vi "MultiGrid_v2.vi"() -> ()   [LabVIEW 2014]
uses:
  <userlib>/Nanonis Prog Interface V5/Nanonis Prog Interface.lvlib
panel:
  out "Y offset":dbl format="%#_6p"
  out "X offset":dbl format="%#_6p"
  in  "Grid":i32(listbox)
  in  "Frame":i32(listbox)
  in  "Cloud Grid":bool=TRUE
  in  "GridSettings":T1={"Imaging Current"=5e-11, "STS Current"=1e-09, "Start value (V)"=-0.05, "End value (V)"=0.05, "Number of points (0=no change)"=256, "File name"="single_mol_shortSTS", "DC pixel"=64.0, "Grid X"=0.0, "Grid Y"=0.0, "Sweeps"=8.0}
  in  "Polling (s)":u32=600
  out "Status":string="Waiting for grid to start"
  out "#Grids":i32=2
  out "MultiGrid":i32(listbox)
  # "0 for no change"
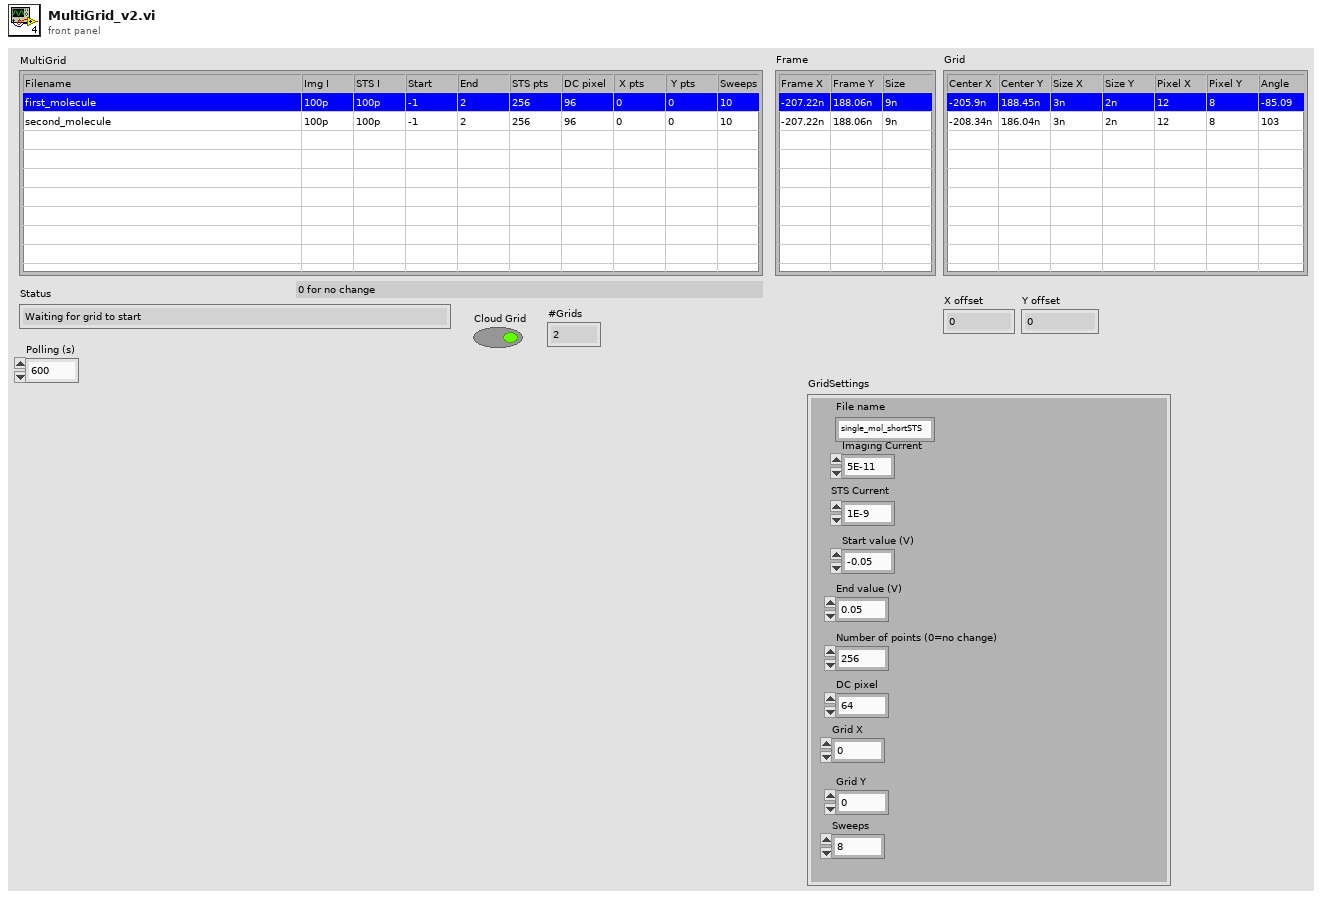
[diagram p1: front panel]
types:
  T1 = cluster{"Imaging Current":sgl, "STS Current":sgl, "Start value (V)":sgl, "End value (V)":sgl, "Number of points (0=no change)":i32, "File name":string, "DC pixel":dbl, "Grid X":dbl, "Grid Y":dbl, "Sweeps":dbl}
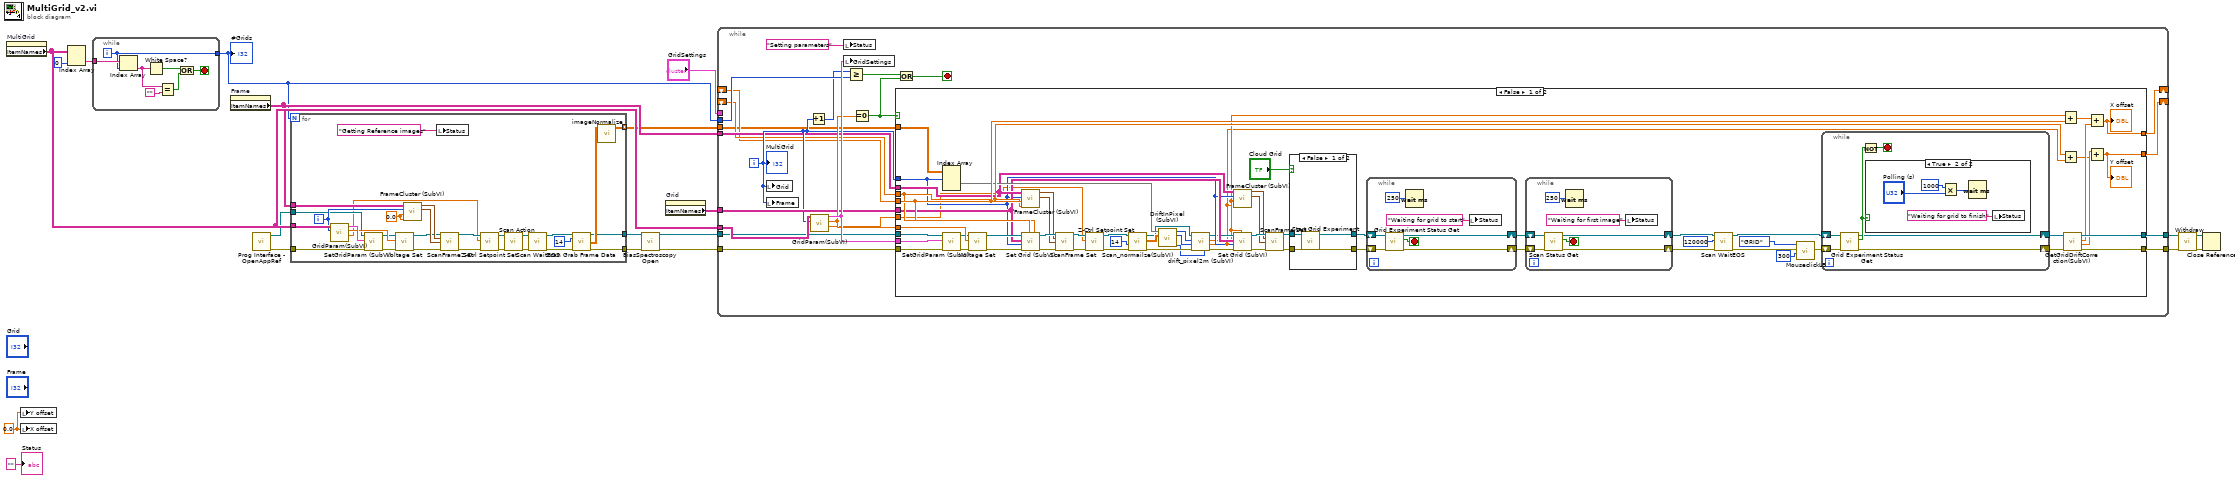
[diagram p0: block diagram]
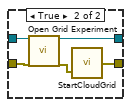
[diagram p2: hidden frame]
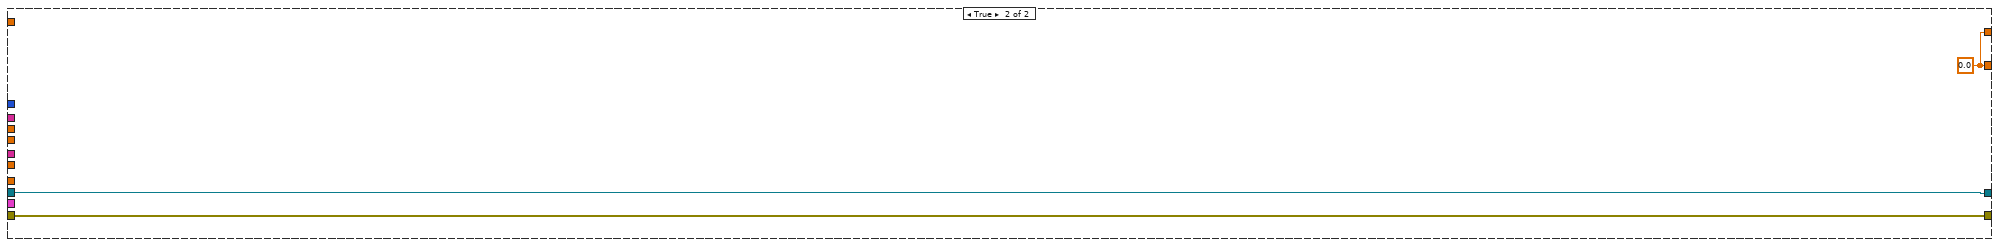
[diagram p4: hidden frame]
diagram:
  w10 = 0.0 ("Y offset")
  n1 = property on="MultiGrid" class="MCListbox (strict)"() -> ("ItemNames"=w8:string[][])  [unwired: 2 in, 2 out]
  n2 = local write "Y offset"(w10) -> ()
  n3 = local write "X offset"(w10) -> ()
  n4 = Index Array(array=w8, index (col)=0 ("disabled index (col)")) -> (element=w17:string[])  [unwired: 1 in]
  n5 = while {
    tunnel: w17 -> [w27]
    tunnel: [w21] -> w2
    i -> [w21]
    stop <- w23 stop-if-true
    n6 = Index Array(array=w27, index=w21) -> (element=w26:string)
    n7 = White Space?(1:w26) -> (0:w24:bool)
    n8 = Equal?(x=w26, y="") -> (x = y?=w22:bool)
    n9 = Or(x=w24, y=w22) -> (x .or. y?=w23:bool)
  }
  "#Grids" <- w2
  n10 = property on="Frame" class="MCListbox (strict)"() -> ("ItemNames"=w7:string[][])  [unwired: 2 in, 2 out]
  n11 = call <userlib>:"Prog Interface - OpenAppRef.vi"() -> ("Error out"=w5:errorcluster, "Application reference"=w6:refnum<vi>)  [unwired: 6 in]
  n12 = for {
    N: w2 -> [_]
    tunnel: w8 -> [w53]
    tunnel: w7 -> [w50]
    tunnel: w6 -> [w45]
    tunnel: w5 -> [w44]
    tunnel: [w36] -> w4
    tunnel: [w35] -> w3
    tunnel: [w33] -> w1 mode=indexing
    i -> [w48]
    w49 = 0.0 ("x offset")
    n13 = call "GridParam(SubVI).vi"("Numeric in"=w48, "ItemNames"=w53) -> ("Img Current"=w28:dbl, "Bias"=w51:dbl, "GridSettings"=w52:T1)  [unwired: 7 in]
    n14 = call "SetGridParam (SubVI).vi"("error in (no error)"=w44, "GridSettings"=w52, "Application in"=w45) -> ("Error out"=w43:errorcluster, "Application ref out"=w42:refnum<vi>)  [unwired: 7 in]
    n15 = call <userlib>:"Voltage Set.vi"("Error in (no error)"=w43, "Bias (V)"=w51, "Application ref in"=w42) -> ("Error out"=w40:errorcluster, "Application ref out"=w41:refnum<vi>)  [unwired: 7 in]
    n16 = call "FrameCluster (SubVI).vi"("y offset"=w49, "x offset"=w49, "index (row)"=w48, "ItemNames"=w50) -> ("Size (m)"=w47:cluster{"Width":sgl, "Height":sgl}, "Center coordinates (m)"=w46:cluster{"Xc":sgl, "Yc":sgl})  [unwired: 6 in]
    n17 = local write "Status"("Getting Reference images" ("Status")) -> ()
    n18 = call <userlib>:"ScanFrame Set.vi"("Application ref in"=w41, "Center coordinates (m)"=w46, "Size (m)"=w47, "error in (no error)"=w40) -> ("Application ref out"=w32:refnum<vi>, "error out"=w31:errorcluster)  [unwired: 10 in]
    n19 = call <userlib>:"Z-Ctrl Setpoint Set.vi"("error in (no error)"=w31, "Z Controller setpoint"=w28, "Application ref in"=w32) -> ("error out"=w29:errorcluster, "Application ref out"=w30:refnum<vi>)  [unwired: 7 in]
    n20 = call <userlib>:"Scan Action.vi"("error in (no error)"=w29, "Application ref in"=w30) -> ("error out"=w39:errorcluster, "Application ref out"=w56:refnum<vi>)  [unwired: 7 in]
    n21 = call <userlib>:"Scan WaitEOS.vi"("error in (no error)"=w39, "Application ref in"=w56) -> ("error out"=w38:errorcluster, "Application ref out"=w55:refnum<vi>)  [unwired: 5 in, 2 out]
    n22 = call <userlib>:"Scan Grab Frame Data.vi"("Application ref in"=w55, "Channel index (0-23)"=u8 14, "error in (no error)"=w38) -> ("Application ref out"=w36:refnum<vi>, "Scan frame data"=w54:sgl[][], "error out"=w35:errorcluster)  [unwired: 8 in, 2 out]
    n23 = call "imageNormalize.vi"("Data"=w54) -> ("Array"=w33:dbl[][])  [unwired: 10 in]
  }
  n24 = call <userlib>:"BiasSpectroscopy Open.vi"("Application ref in"=w4, "Error in (no error)"=w3) -> ("Application ref out"=w12:refnum<vi>, "Error out"=w11:errorcluster)  [unwired: 12 in]
  n25 = property on="Grid" class="MCListbox (strict)"() -> ("ItemNames"=w9:string[][])  [unwired: 2 in, 2 out]
  n26 = while {
    tunnel: w8 -> [w78]
    tunnel: w12 -> [w72]
    tunnel: w11 -> [w71]
    tunnel: "GridSettings" -> [_]
    tunnel: [w70] -> w20
    tunnel: [w73] -> w19
    tunnel: w2 -> [w74]
    shift-right: [w65] -> _
    shift-left: _ -> [w59]
    shift-right: [w64] -> _
    shift-left: _ -> [w60]
    tunnel: w9 -> [w63]
    tunnel: w7 -> [w61]
    tunnel: w1 -> [w58]
    i -> [w62]
    stop <- w69 stop-if-true
    n27 = local write "Grid"(w62) -> ()
    n28 = local write "Frame"(w62) -> ()
    n29 = Increment(x=w62) -> (x+1=w68:i32)
    n30 = call "GridParam(SubVI).vi"("Numeric in"=w62, "ItemNames"=w78) -> ("Img Current"=w57:dbl, "Bias"=w66:dbl, "GridSettings"=w77:T1)  [unwired: 7 in]
    n31 = local write "Status"("Setting parameters" ("Status")) -> ()
    n32 = local write "GridSettings"(w77) -> ()
    n33 = Greater Or Equal?(x=w68, y=w74) -> (x >= y?=w75:bool)
    n34 = Equal To 0?(x=w66) -> (x = 0?=w67:bool)
    n35 = case shown="False" w67 {
      tunnel: w77 -> [w142 _]
      tunnel: [w120 w177] -> w73
      tunnel: w72 -> [w141 w178]
      tunnel: w71 -> [w140 w177]
      tunnel: [w122 w178] -> w70
      tunnel: w66 -> [w126 _]
      tunnel: [w110 w176] -> w65
      tunnel: [w111 w176] -> w64
      tunnel: w63 -> [w93 _]
      tunnel: w62 -> [w92 _]
      tunnel: w61 -> [w94 _]
      tunnel: w60 -> [w108 _]
      tunnel: w59 -> [w109 _]
      tunnel: w58 -> [w101 _]
      tunnel: w57 -> [w79 _]
      frame False {
        n36 = Index Array(array=w101, index (dim 0)=w92) -> (element=w100:dbl[][])  [unwired: 2 in]
        n37 = call "SetGridParam (SubVI).vi"("error in (no error)"=w140, "GridSettings"=w142, "Application in"=w141) -> ("Error out"=w124:errorcluster, "Application ref out"=w125:refnum<vi>)  [unwired: 7 in]
        n38 = call <userlib>:"Voltage Set.vi"("Error in (no error)"=w124, "Bias (V)"=w126, "Application ref in"=w125) -> ("Error out"=w112:errorcluster, "Application ref out"=w117:refnum<vi>)  [unwired: 7 in]
        n39 = call "FrameCluster (SubVI).vi"("y offset"=w108, "x offset"=w109, "index (row)"=w92, "ItemNames"=w94) -> ("Size (m)"=w114:cluster{"Width":sgl, "Height":sgl}, "Center coordinates (m)"=w115:cluster{"Xc":sgl, "Yc":sgl})  [unwired: 6 in]
        n40 = call "Set Grid (SubVI).vi"("y offset"=w108, "x offset"=w109, "error in (no error)"=w112, "index (row)"=w92, "ItemNames"=w93, "Application in"=w117) -> ("error out"=w113:errorcluster, "Application out"=w116:refnum<vi>)  [unwired: 4 in]
        n41 = call <userlib>:"ScanFrame Set.vi"("Application ref in"=w116, "Center coordinates (m)"=w115, "Size (m)"=w114, "error in (no error)"=w113) -> ("Application ref out"=w107:refnum<vi>, "error out"=w106:errorcluster)  [unwired: 10 in]
        n42 = call <userlib>:"Z-Ctrl Setpoint Set.vi"("error in (no error)"=w106, "Z Controller setpoint"=w79, "Application ref in"=w107) -> ("error out"=w104:errorcluster, "Application ref out"=w105:refnum<vi>)  [unwired: 7 in]
        n43 = call "Scan_normailze(SubVI).vi"("error in (no error)"=w104, "Channel index (0-23)"=u8 14, "Application in"=w105) -> ("error out"=w98:errorcluster, "Array"=w102:dbl[][], "Application out"=w99:refnum<vi>)  [unwired: 6 in]
        n44 = call "DriftInPixel (SubVI).vi"("New image"=w102, "Ref image"=w100) -> ("pixel"=w97:i32, "Y drift"=w95:i32, "X drift"=w96:i32)  [unwired: 7 in]
        n45 = call "drift_pixel2m (SubVI).vi"("Application in"=w99, "X drift"=w96, "Y drift"=w95, "error in"=w98, "Drift correction Pixels"=w97) -> ("Application out"=w91:refnum<vi>, "x drift"=w81:sgl, "y drift"=w80:sgl, "error out"=w90:errorcluster)  [unwired: 1 in]
        n46 = call "FrameCluster (SubVI).vi"("y offset"=w80, "x offset"=w81, "index (row)"=w92, "ItemNames"=w94) -> ("Size (m)"=w86:cluster{"Width":sgl, "Height":sgl}, "Center coordinates (m)"=w87:cluster{"Xc":sgl, "Yc":sgl})  [unwired: 6 in]
        n47 = call "Set Grid (SubVI).vi"("y offset"=w80, "x offset"=w81, "error in (no error)"=w90, "index (row)"=w92, "ItemNames"=w93, "Application in"=w91) -> ("error out"=w89:errorcluster, "Application out"=w88:refnum<vi>)  [unwired: 4 in]
        n48 = call <userlib>:"ScanFrame Set.vi"("Application ref in"=w88, "Center coordinates (m)"=w87, "Size (m)"=w86, "error in (no error)"=w89) -> ("Application ref out"=w85:refnum<vi>, "error out"=w84:errorcluster)  [unwired: 10 in]
        n49 = case shown="False" "Cloud Grid" {
          tunnel: w84 -> [w160 w163]
          tunnel: [w159 w164] -> w138
          tunnel: [w158 w162] -> w137
          tunnel: w85 -> [w157 w165]
          frame False {
            n50 = call <userlib>:"Start Grid Experiment.vi"("Application ref in"=w157, "error in (no error)"=w160) -> ("Application ref out"=w159:refnum<vi>, "error out"=w158:errorcluster)  [unwired: 16 in]
          }
          frame True {
            n51 = call <userlib>:"Open Grid Experiment.vi"("Application ref in"=w165, "error in (no error)"=w163) -> ("Application ref out"=w164:refnum<vi>, "error out"=w161:errorcluster)  [unwired: 16 in]
            n52 = call "StartCloudGrid.vi"("error in (no error)"=w161) -> ("error out"=w162:errorcluster)  [unwired: 1 in]
          }
        }
        n53 = while {
          shift-right: [w156] -> w131
          shift-left: w138 -> [w152]
          shift-right: [w151] -> w127
          shift-left: w137 -> [w155]
          stop <- w150 stop-if-true
          n54 = call <userlib>:"Grid Experiment Status Get.vi"("error in (no error)"=w155, "Application ref in"=w152) -> ("error out"=w151:errorcluster, "Running?"=w150:bool, "Application ref out"=w156:refnum<vi>)  [unwired: 7 in]
          n55 = Wait (ms)(milliseconds to wait=u32 250) -> ()  [unwired: 1 out]
          n56 = local write "Status"("Waiting for grid to start" ("Status")) -> ()
        }
        n57 = while {
          shift-right: [w147] -> w130
          shift-left: w131 -> [w148]
          shift-right: [w146] -> w129
          shift-left: w127 -> [w149]
          stop <- w145 stop-if-true
          n58 = call <userlib>:"Scan Status Get.vi"("error in (no error)"=w149, "Application ref in"=w148) -> ("error out"=w146:errorcluster, "Scanning?"=w145:bool, "Application ref out"=w147:refnum<vi>)  [unwired: 6 in]
          n59 = Wait (ms)(milliseconds to wait=u32 250) -> ()  [unwired: 1 out]
          n60 = local write "Status"("Waiting for first image" ("Status")) -> ()
        }
        n61 = call <userlib>:"Scan WaitEOS.vi"("error in (no error)"=w129, "Timeout in ms (-1)"=120000, "Application ref in"=w130) -> ("error out"=w133:errorcluster, "Application ref out"=w132:refnum<vi>)  [unwired: 4 in, 2 out]
        n62 = call "MouseclickLB.vi"("nMilliseconds"=300, "error in (no error)"=w133, "Click"=enum16{"Header", "TOPO", "STS", "GRID"}."GRID") -> ("error out"=w136:errorcluster)  [unwired: 8 in]
        n63 = while {
          shift-right: [w168] -> w123
          shift-left: w132 -> [w169]
          shift-right: [w166] -> w121
          shift-left: w136 -> [w167]
          stop <- w171 stop-if-true
          n64 = call <userlib>:"Grid Experiment Status Get.vi"("error in (no error)"=w167, "Application ref in"=w169) -> ("error out"=w166:errorcluster, "Running?"=w170:bool, "Application ref out"=w168:refnum<vi>)  [unwired: 7 in]
          n65 = Not(x=w170) -> (.not. x?=w171:bool)
          n66 = case shown="True" w170 {
            frame False {
            }
            frame True {
              n67 = Multiply(x=u32 1000, y="Polling (s)") -> (x*y=w174:u32)
              n68 = Wait (ms)(milliseconds to wait=w174) -> ()  [unwired: 1 out]
              n69 = local write "Status"("Waiting for grid to finish" ("Status")) -> ()
            }
          }
        }
        n70 = Add(x=w81, y=w109) -> (x+y=w83:dbl)
        n71 = Add(x=w108, y=w80) -> (x+y=w82:dbl)
        n72 = call "GetGridDriftCorrection(SubVI).vi"("error in (no error)"=w121, "Application in"=w123) -> ("Error out"=w120:errorcluster, "Y offset"=w118:dbl, "X offset"=w119:dbl, "Application ref out"=w122:refnum<vi>)  [unwired: 6 in]
        n73 = Add(x=w83, y=w119) -> (x+y=w110:dbl)
        "X offset" <- w110
        n74 = Add(x=w118, y=w82) -> (x+y=w111:dbl)
        "Y offset" <- w111
      }
      frame True {
        w176 = 0.0 ("X offset")
      }
    }
    n75 = Or(x=w75, y=w67) -> (x .or. y?=w69:bool)
    "MultiGrid" <- w62
  }
  n76 = call <userlib>:"Withdraw.vi"("Error in (no error)"=w19, "Application ref in"=w20) -> ("Error out"=w13:errorcluster, "Application ref out"=w14:refnum<vi>)  [unwired: 8 in]
  n77 = Close Reference(reference=w14, error in (no error)=w13) -> ()  [unwired: 1 out]
  "Status" <- "" ("Status")
